vi "Savitzky-Golay Filter (DBL).vi"(8 "Weight":dbl[](array[numeric]), 9 "polynomial order":i32=3, 10 "side points":i32=6, 11 "X":dbl[](array[numeric])) -> (0 "error":i32, 3 "Filtered X":dbl[](array[numeric]))   [LabVIEW 2024, in "NI_AALBase.lvlib"]
doc: "<p>Filters the input data sequence<strong> X</strong> using a Savitzky-Golay FIR smoothing filter. Wire data to the <strong>X</strong> input to determine the polymorphic instance to use or <a href=\"nihelplauncher://docs/csh?context=lvcore_lvhowto_selectingdefaultinstpolyvi\">manually select</a> the instance.\n</p>"
uses:
  NI_AALBase.lvlib
  <resource>/lvanlys.dll
panel:
  # "Savitzky-Golay Filter"
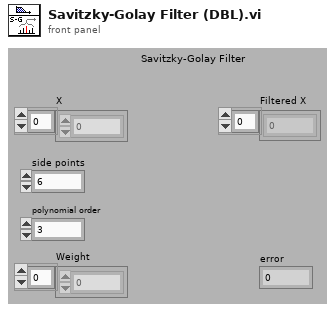
[diagram p1: front panel]
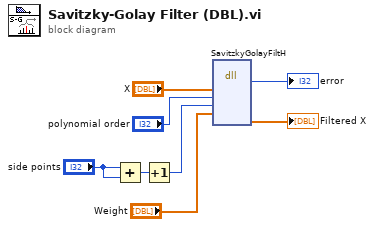
[diagram p0: block diagram]
diagram:
  n1 = Add(x="side points", y="side points") -> (x+y=w3:i32)
  n2 = Increment(x=w3) -> (x+1=w1:i32)
  n3 = dll-call lib="C:/Program Files (x86)/National Instruments/LabVIEW 2024/resource/lvanlys.*" fn="SavitzkyGolayFiltH"("xH"="X", "polyOrder"="polynomial order", "frameSize"=w1, "weight"="Weight") -> (→"error":i32, "yH"=→"Filtered X":dbl[])  [unwired: 8 in, 2 out]
